vi "波形数组.vi"() -> ()   [LabVIEW 2015]
uses:
  <vilib>/Waveform/WDTOps.llb/WDT Index Channel DBL.vi
  <vilib>/Waveform/WDTOps.llb/WDT Index Channel by Name DBL.vi
  <vilib>/measure/NI_MABase.lvlib
panel:
  out "合并波形":dynamicdata(graph)
  out "Waveform Graph":waveform(dbl)(graph)
  in  "波形索引":dbl
  out "索引波形图":waveform(dbl)(graph)
  out "波形数据数组":waveform(dbl)[](array[waveform])
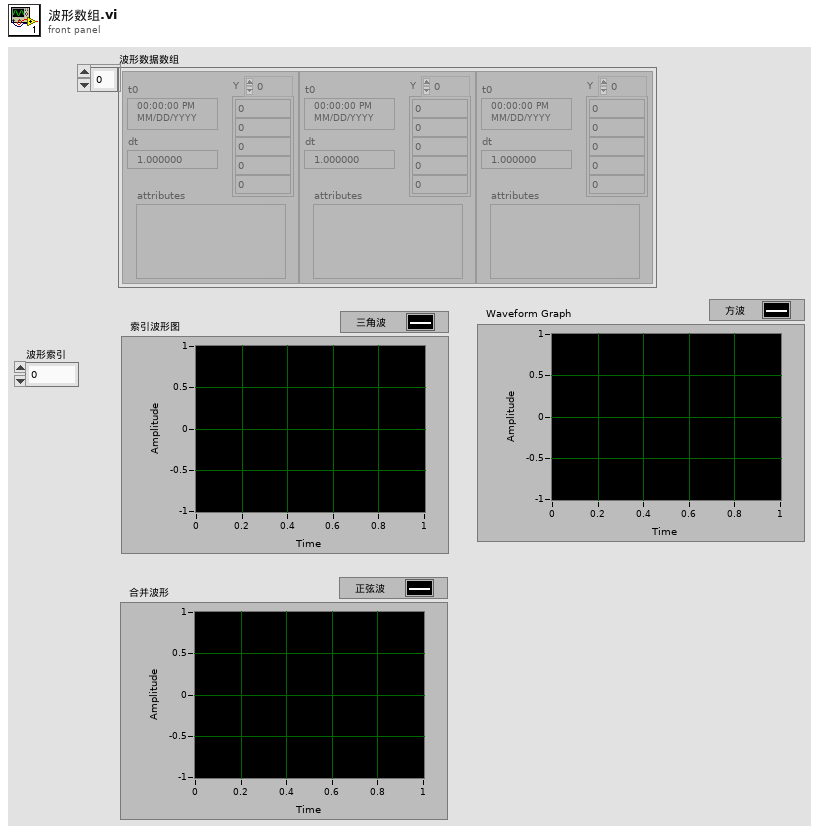
[diagram p1: front panel]
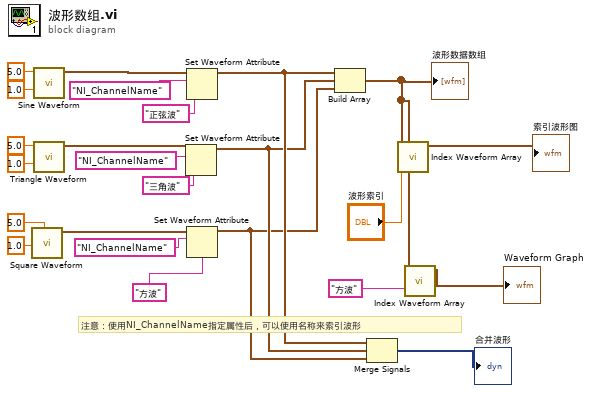
[diagram p0: block diagram]
diagram:
  # "注意：使用NI_ChannelName指定属性后，可以使用名称来索引波形"
  n1 = call <vilib>:"Square Waveform.vi"("amplitude"=1.0, "frequency"=5.0) -> ("signal out"=w10:waveform(dbl))  [unwired: 8 in, 1 out]
  n2 = call <vilib>:"Sine Waveform.vi"("amplitude"=1.0, "frequency"=5.0) -> ("signal out"=w18:waveform(dbl))  [unwired: 8 in, 1 out]
  n3 = call <vilib>:"Triangle Waveform.vi"("amplitude"=1.0, "frequency"=5.0) -> ("signal out"=w15:waveform(dbl))  [unwired: 8 in, 1 out]
  n4 = Set Waveform Attribute(5:"三角波", 6:"NI_ChannelName" ("name"), 7:w15) -> (3:w3:waveform(dbl))  [unwired: 1 in, 2 out]
  n5 = Set Waveform Attribute(5:"正弦波", 6:"NI_ChannelName" ("name"), 7:w18) -> (3:w4:waveform(dbl))  [unwired: 1 in, 2 out]
  n6 = Set Waveform Attribute(5:"方波" ("value"), 6:"NI_ChannelName" ("name"), 7:w10) -> (3:w2:waveform(dbl))  [unwired: 1 in, 2 out]
  n7 = Build Array(w4, w3, w2) -> (w6:waveform(dbl)[])
  "波形数据数组" <- w6
  n8 = Merge Signals(w4, w3, w2) -> (→"合并波形":dynamicdata)
  n9 = call-poly <vilib>:"Index Waveform Array.vi"("index"="波形索引", "waveform array"=w6) -> ("waveform"=→"索引波形图":waveform(dbl))  [unwired: 8 in, 1 out]
  n10 = call-poly <vilib>:"Index Waveform Array.vi"("channel name"="方波", "waveform array"=w6) -> ("waveform"=→"Waveform Graph":waveform(dbl))  [unwired: 8 in, 1 out]
